vi "Particle Analysis Report.vi"() -> ()   [LabVIEW 2015]
doc: "This example introduces the processing area of particle analysis. This example uses the threshold function that converts a grayscale image into a binary image."
uses:
  <vilib>/vision/NI_Vision_Development_Module.lvlib
panel:
  in  "Stop":bool
  out "Selected Particle Report":T1 {"Orientation" format="%.2f"; "Center of Mass"."Y" format="%.2f"; "Center of Mass"."X" format="%.2f"}
  in  "Selected Particle":i32(slide)=2 min=-3 max=0
  out "Threshold Image":T2(plugin-control)
  # "Overview: Demonstrates how to use the IMAQ Particle Analysis Report function with a binary image to return information about each particle.\nRequirements: Vision Development Software.\nInstructions:\n1. Run the VI.\n2. Change the Selected Particle to update the Selected Particle Report, and overlay the bounding box for the selected particle."
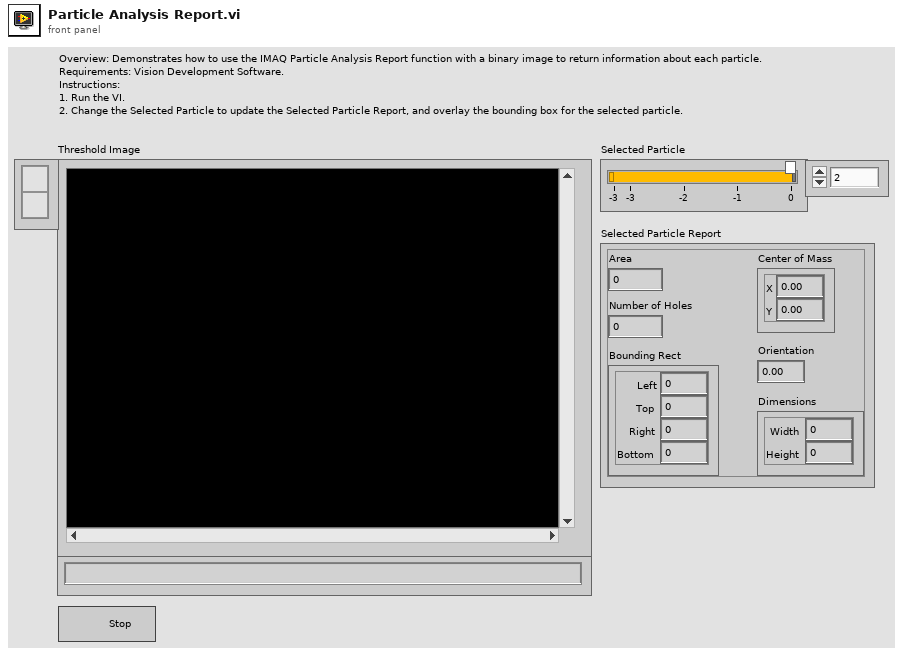
[diagram p1: front panel]
types:
  T1 = cluster{"Area":dbl, "Number of Holes":dbl, "Bounding Rect":cluster{"Left":dbl, "Top":dbl, "Right":dbl, "Bottom":dbl}, "Center of Mass":cluster{"X":dbl, "Y":dbl}, "Orientation":dbl, "Dimensions":cluster{"Width":dbl, "Height":dbl}}
  T2 = typedef "IMAQ Image.ctl" = refnum<image>
  T3 = cluster{"Area":dbl, "Number of Holes":dbl, "Bounding Rect":cluster{"Left":dbl, "Top":dbl, "Right":dbl, "Bottom":dbl}, "Center of Mass":cluster{"X":dbl, "Y":dbl}, "Orientation":dbl, "Dimensions":cluster{"Width":dbl, "Height":dbl}}[]
  T4 = cluster{"Left":dbl, "Top":dbl, "Right":dbl, "Bottom":dbl}
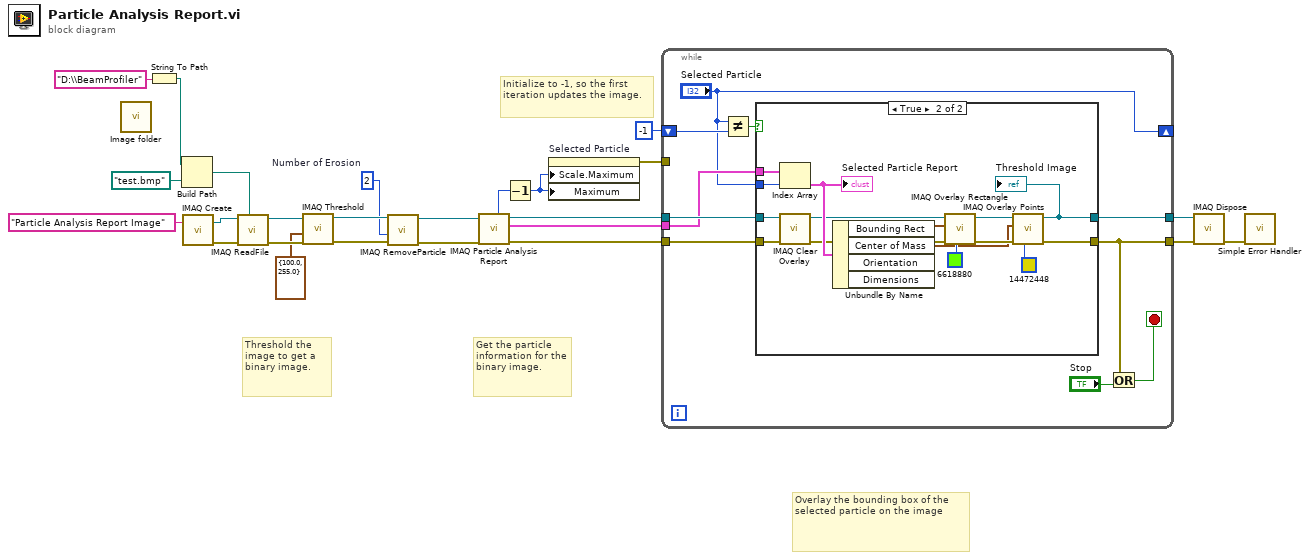
[diagram p0: block diagram]
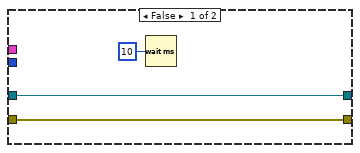
[diagram p2: hidden frame]
diagram:
  w1 = 2  # Number of Erosion
  # "Initialize to -1, so the first iteration updates the image."
  # "Overlay the bounding box of the selected particle on the image"
  # "Get the particle information for the binary image."
  # "Threshold the image to get a binary image."
  n1 = call "Image folder.vi"() -> ()  [unwired: 11 in, 1 out]
  n2 = String To Path(string="D:\\BeamProfiler" ("Image Name")) -> (path=w6:path)
  n3 = Build Path(base path=w6, name or relative path=path "test.bmp") -> (appended path=w21:path)
  n4 = call "IMAQ Create"("Image Name"="Particle Analysis Report Image") -> ("New Image"=w24:T2, "error out"=w23:errorcluster)  [unwired: 4 in]
  n5 = call "IMAQ ReadFile"("File Path"=w21, "error in (no error)"=w23, "Image"=w24) -> ("error out"=w19:errorcluster, "Image Out"=w20:T2)  [unwired: 4 in, 3 out]
  n6 = call "IMAQ Threshold"("error in (no error)"=w19, "Range"=cluster{"Lower value":sgl, "Upper value":sgl} {"Lower value"=100.0, "Upper value"=255.0}, "Image Src"=w20) -> ("error out"=w4:errorcluster, "Image Dst Out"=w5:T2)  [unwired: 7 in]
  n7 = call "IMAQ RemoveParticle"("error in (no error)"=w4, "Number of Erosion"=w1, "Image Src"=w5) -> ("error out"=w3:errorcluster, "Image Dst Out"=w2:T2)  [unwired: 7 in]
  n8 = call "IMAQ Particle Analysis Report"("error in (no error)"=w3, "Image"=w2) -> ("error out"=w16:errorcluster, "Particle Reports (Pixels)"=w13:T3, "Image Out (duplicate)"=w17:T2, "Number of Particles"=w14:i32)  [unwired: 4 in, 2 out]
  n9 = Decrement(x=w14) -> (x-1=w10:i32)
  n10 = property on="Selected Particle" class="Slide (strict)"("Scale.Maximum"=w10, "Maximum"=w10) -> (error out=w9:errorcluster)  [unwired: 2 in, 1 out]
  n11 = while {
    tunnel: w17 -> [w35]
    tunnel: w16 -> [w34]
    tunnel: [w28] -> w15
    tunnel: [w33] -> w12
    tunnel: w13 -> [w31]
    shift-right: ["Selected Particle"] -> _
    shift-left: -1 ("Selected Particle") -> [w32]
    tunnel: w9 -> [_]
    stop <- w27 stop-if-true
    n12 = Not Equal?(x="Selected Particle", y=w32) -> (x != y?=w30:bool)
    n13 = case shown="True" w30 {
      tunnel: w35 -> [w38 w49]
      tunnel: w34 -> [w37 w48]
      tunnel: [w37 w43] -> w28
      tunnel: [w38 w40] -> w33
      tunnel: w31 -> [_ w51]
      tunnel: "Selected Particle" -> [_ w45]
      frame False {
        n14 = Wait (ms)(milliseconds to wait=u32 10) -> ()  [unwired: 1 out]
      }
      frame True {
        n15 = Index Array(array=w51, index=w45) -> (element=w50:T1)
        "Selected Particle Report" <- w50
        n16 = call "IMAQ Clear Overlay"("error in (no error)"=w48, "Image"=w49) -> ("error out"=w46:errorcluster, "Image Out"=w47:T2)  [unwired: 8 in]
        n17 = Unbundle By Name(w50) -> ("Bounding Rect"=w53:T4, "Center of Mass"=w41:cluster{"X":dbl, "Y":dbl})  [unwired: 2 out]
        n18 = call "IMAQ Overlay Rectangle"("Color"=u32 6618880, "error in (no error)"=w46, "Rectangle"=w53, "Image"=w47) -> ("error out"=w42:errorcluster, "Image Out"=w44:T2)  [unwired: 6 in]
        n19 = call "IMAQ Overlay Points"("Color"=u32 14472448, "error in (no error)"=w42, "Point"=w41, "Image"=w44) -> ("error out"=w43:errorcluster, "Image Out"=w40:T2)  [unwired: 6 in]
        "Threshold Image" <- w40
      }
    }
    n20 = Or(x=w28, y="Stop") -> (x .or. y?=w27:bool)
  }
  n21 = call "IMAQ Dispose"("Image"=w12, "error in (no error)"=w15) -> ("error out"=w18:errorcluster)  [unwired: 4 in]
  n22 = call <vilib>:"Simple Error Handler.vi"("error in (no error)"=w18) -> ()  [unwired: 4 in, 5 out]
